vi "Two Ball.vi"() -> ()   [LabVIEW 2014]
uses:
  Team Code/Robot Global Data.vi
panel:
  in  "Loops to wait before Firing":i32=10
  out "Angle":dbl
  out "Distance (in)":dbl
  in  "Min. Power":dbl=0.1 format="%#_13g"
  in  "Roller / Drive Ratio":dbl=1.0
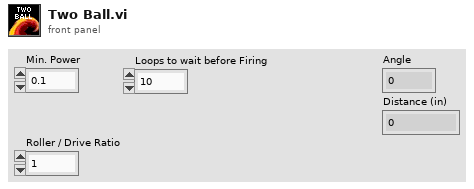
[diagram p1: front panel]
types:
  T1 = cluster{"FIRE!!!":bool, "Loader":bool, "Lock":bool, "Load":bool, "Pass":bool, "Grab":bool, "PANIC":bool, "Don't Cock":bool, "Roller Speed":dbl}
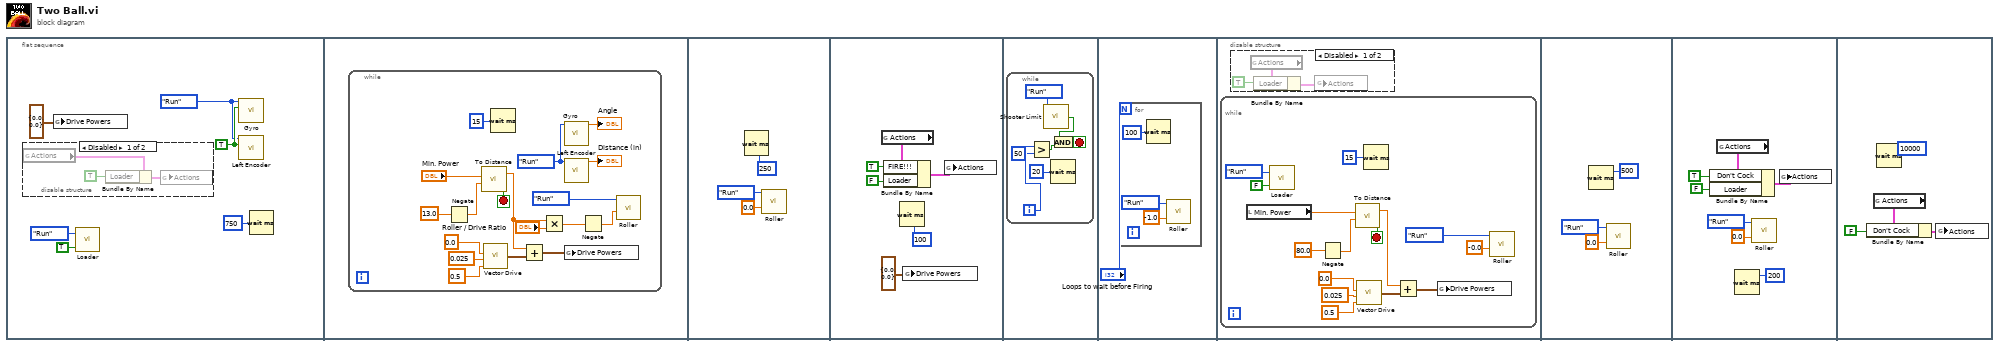
[diagram p0: block diagram]
diagram:
  n1 = flat-sequence {
    frame #0 {
      w5 = enum16{"Start", "Run", "End"}."Run" ("Enum")
      w6 = TRUE ("Reset")
      n2 = disable-structure shown="Disabled" {
        frame Disabled {
          n3 = global read "Robot Global Data.vi" "Actions"() -> (w8:T1)
          n4 = Bundle By Name(cluster=w8, "Loader"=TRUE ("Primary Action")) -> (w9:T1)
          n5 = global write "Robot Global Data.vi" "Actions"(w9) -> ()
        }
        frame Enabled {
        }
      }
      n6 = global write "Robot Global Data.vi" "Drive Powers"(cluster{"Right":dbl, "Left":dbl} {"Right"=0.0, "Left"=0.0} ("Drive Powers")) -> ()
      n7 = call "Loader.vi"("Down (Forward)"=TRUE, "Enum"=enum16{"Start", "Run", "End"}."Run") -> ()  [unwired: 1 out]
      n8 = call "Gyro.vi"("Reset"=w6, "Enum"=w5) -> ()  [unwired: 9 in, 1 out]
      n9 = call "Left Encoder.vi"("Reset"=w6, "Enum"=w5) -> ()  [unwired: 8 in, 2 out]
      n10 = Wait (ms)(milliseconds to wait=u32 750) -> ()  [unwired: 1 out]
    }
    frame #1 {
      n11 = while {
        stop <- w26 stop-if-true
        w19 = enum16{"Start", "Run", "End"}."Run" ("Enum")
        n12 = Negate(x=13.0) -> (-x=w17:dbl)
        n13 = call "To Distance.vi"("Destination Dist (in)"=w17, "Min. Power"="Min. Power") -> ("Reached Distance"=w26:bool, "Base Speed"=w15:dbl)  [unwired: 2 in]
        n14 = call "Vector Drive.vi"("Tolerance"=0.5, "Min. Power"=0.025, "Angle"=0.0) -> ("Motor Powers"=w22:cluster{"RMotor":dbl, "LMotor":dbl})  [unwired: 1 in]
        n15 = Wait (ms)(milliseconds to wait=u32 15) -> ()  [unwired: 1 out]
        n16 = Add(x=w15, y=w22) -> (x+y=w21:cluster{"RMotor":dbl, "LMotor":dbl})
        n17 = Multiply(x=w15, y="Roller / Drive Ratio") -> (x*y=w12:dbl)
        n18 = call "Gyro.vi"("Enum"=w19) -> ("Angle"=→"Angle":dbl)  [unwired: 10 in]
        n19 = call "Left Encoder.vi"("Enum"=w19) -> ("Distance (in)"=→"Distance (in)":dbl)  [unwired: 9 in, 1 out]
        n20 = global write "Robot Global Data.vi" "Drive Powers"(w21) -> ()
        n21 = Negate(x=w12) -> (-x=w11:dbl)
        n22 = call "Roller.vi"("Power"=w11, "Enum"=enum16{"Start", "Run", "End"}."Run") -> ()  [unwired: 2 in]
      }
    }
    frame #2 {
      n23 = Wait (ms)(milliseconds to wait=u32 250) -> ()  [unwired: 1 out]
      n24 = call "Roller.vi"("Power"=0.0, "Enum"=enum16{"Start", "Run", "End"}."Run") -> ()  [unwired: 2 in]
    }
    frame #3 {
      n25 = global read "Robot Global Data.vi" "Actions"() -> (w35:T1)
      n26 = Bundle By Name(cluster=w35, "FIRE!!!"=TRUE ("Primary Action"), "Loader"=FALSE) -> (w36:T1)
      n27 = Wait (ms)(milliseconds to wait=u32 100) -> ()  [unwired: 1 out]
      n28 = global write "Robot Global Data.vi" "Drive Powers"(cluster{"Right":dbl, "Left":dbl} {"Right"=0.0, "Left"=0.0} ("Drive Powers")) -> ()
      n29 = global write "Robot Global Data.vi" "Actions"(w36) -> ()
    }
    frame #4 {
      n30 = while {
        i -> [w40]
        stop <- w37 stop-if-true
        n31 = Greater?(x=w40, y=50) -> (0:w38:bool)
        n32 = call "Shooter Limit.vi"("Enum"=enum16{"Start", "Run", "End"}."Run") -> ("Value"=w41:bool)  [unwired: 1 in]
        n33 = Wait (ms)(milliseconds to wait=u32 20) -> ()  [unwired: 1 out]
        n34 = And(x=w41, y=w38) -> (x .and. y?=w37:bool)
      }
    }
    frame #5 {
      n35 = for {
        N: "Loops to wait before Firing" -> [_]
        n36 = Wait (ms)(milliseconds to wait=u32 100) -> ()  [unwired: 1 out]
        n37 = call "Roller.vi"("Power"=-1.0, "Enum"=enum16{"Start", "Run", "End"}."Run") -> ()  [unwired: 2 in]
      }
    }
    frame #6 {
      n38 = while {
        stop <- w65 stop-if-true
        n39 = local read "Min. Power"() -> (w54:dbl)
        n40 = call "Loader.vi"("Down (Forward)"=FALSE, "Enum"=enum16{"Start", "Run", "End"}."Run") -> ()  [unwired: 1 out]
        n41 = Negate(x=80.0) -> (-x=w59:dbl)
        n42 = call "To Distance.vi"("Destination Dist (in)"=w59, "Min. Power"=w54) -> ("Reached Distance"=w65:bool, "Base Speed"=w57:dbl)  [unwired: 2 in]
        n43 = call "Vector Drive.vi"("Tolerance"=0.5, "Min. Power"=0.025, "Angle"=0.0) -> ("Motor Powers"=w61:cluster{"RMotor":dbl, "LMotor":dbl})  [unwired: 1 in]
        n44 = Wait (ms)(milliseconds to wait=u32 15) -> ()  [unwired: 1 out]
        n45 = Add(x=w57, y=w61) -> (x+y=w60:cluster{"RMotor":dbl, "LMotor":dbl})
        n46 = global write "Robot Global Data.vi" "Drive Powers"(w60) -> ()
        n47 = call "Roller.vi"("Power"=-0.0, "Enum"=enum16{"Start", "Run", "End"}."Run") -> ()  [unwired: 2 in]
      }
      n48 = disable-structure shown="Disabled" {
        frame Disabled {
          n49 = global read "Robot Global Data.vi" "Actions"() -> (w49:T1)
          n50 = Bundle By Name(cluster=w49, "Loader"=TRUE) -> (w48:T1)
          n51 = global write "Robot Global Data.vi" "Actions"(w48) -> ()
        }
        frame Enabled {
        }
      }
    }
    frame #7 {
      n52 = Wait (ms)(milliseconds to wait=u32 500) -> ()  [unwired: 1 out]
      n53 = call "Roller.vi"("Power"=0.0, "Enum"=enum16{"Start", "Run", "End"}."Run") -> ()  [unwired: 2 in]
    }
    frame #8 {
      n54 = global read "Robot Global Data.vi" "Actions"() -> (w75:T1)
      n55 = Bundle By Name(cluster=w75, "Don't Cock"=TRUE ("Primary Action"), "Loader"=FALSE) -> (w74:T1)
      n56 = Wait (ms)(milliseconds to wait=u32 200) -> ()  [unwired: 1 out]
      n57 = call "Roller.vi"("Power"=0.0, "Enum"=enum16{"Start", "Run", "End"}."Run") -> ()  [unwired: 2 in]
      n58 = global write "Robot Global Data.vi" "Actions"(w74) -> ()
    }
    frame #9 {
      n59 = global read "Robot Global Data.vi" "Actions"() -> (w76:T1)
      n60 = Bundle By Name(cluster=w76, "Don't Cock"=FALSE ("Primary Action")) -> (w77:T1)
      n61 = Wait (ms)(milliseconds to wait=u32 10000) -> ()  [unwired: 1 out]
      n62 = global write "Robot Global Data.vi" "Actions"(w77) -> ()
    }
  }
